vi "FromRepo.vi"(8 "error in":errorcluster, 9 "from repo cluster":T2, 10 "repository in":refnum<class "NISE_CEF_Repository.lvclass">, 11 "node in":refnum<class "Target.lvclass">) -> (0 "error out":errorcluster, 2 "repository out":refnum<class "NISE_CEF_Repository.lvclass">, 3 "node":T1)   [LabVIEW 2015, in "Target.lvclass"]
doc: "Grabs information from the Repo and stores it in the nodes."
uses:
  Target.lvclass
  <vilib>/NI/Configuration Framework/Repository/NISE_CEF_Repository.lvclass
  <vilib>/NI/Configuration Framework/Node/FromRepoCluster.ctl
  <vilib>/NI/Configuration Framework/Node/NodeRef.ctl
  <vilib>/NI/Configuration Framework/Node/NISE_CEF_Node.lvclass
  CustomDeviceRepo/CustomDeviceRepo.lvclass
  CustomDeviceRepo/CustomDeviceRepo.lvclass/CustomDeviceRepo.ctl
  Target.lvclass/Target.ctl
  CustomDeviceRepo/Read Supported Targets Properties.vi
  Write Source.vi
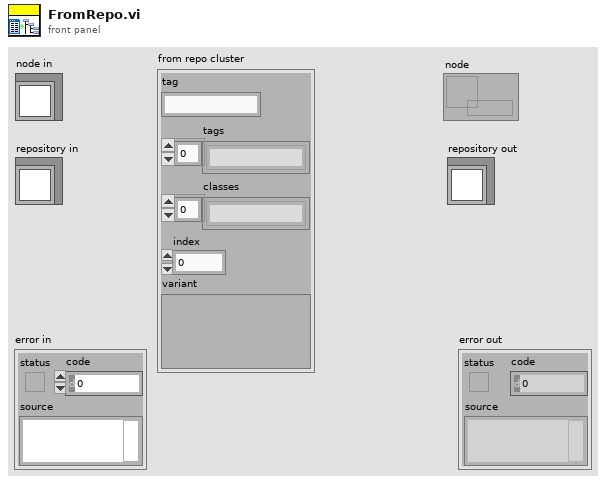
[diagram p1: front panel]
types:
  T1 = typedef "NISE_CEF_Node.lvclass/NodeRef.ctl" = refnum<data-value>
  T2 = typedef "NISE_CEF_Node.lvclass/FromRepoCluster.ctl" = cluster{"tag":string, "tags":string[], "classes":string[], "index":i32, "variant":variant}
  T3 = typedef "Source Distribution for Custom Device VI.ctl" = cluster{"Source":T4, "Real Time System Destination":string, "Supported Target":T5}[]
  T4 = typedef "Path Cluster.ctl" = cluster{"Path":path, "Path Type":enum16{"Absolute", "To Base", "To Common Doc Dir", "To Application Data Dir"}}
  T5 = typedef "Target.ctl" = enum16{"All", "Pharlap", "VxWorks", "Windows", "Linux_32_ARM", "Linux_x64", "PharlapWindows", "PharlapVxWorks", "VxWorksWindows"}
  T6 = cluster{"Source":T4, "Real Time System Destination":string, "Supported Target":T5}
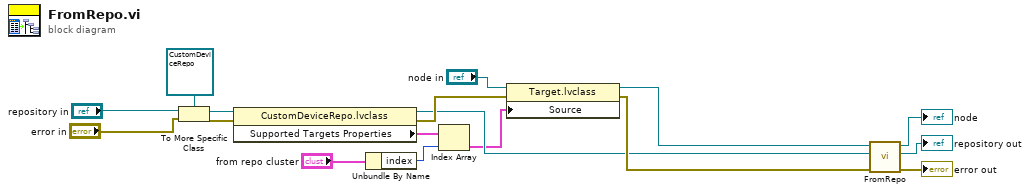
[diagram p0: block diagram]
diagram:
  n1 = To More Specific Class(target class=refnum<class "CustomDeviceRepo.lvclass"> refnum, reference="repository in", error in="error in") -> (specific class reference=w10:refnum<class "CustomDeviceRepo.lvclass">, error out=w8:errorcluster)
  n2 = property class="CustomDeviceRepo.lvclass"(reference=w10, error in=w8) -> (reference out=w2:refnum<class "CustomDeviceRepo.lvclass">, error out=w5:errorcluster, "Supported Targets Properties"=w7:T3)
  n3 = Unbundle By Name("from repo cluster") -> ("index"=w6:i32)
  n4 = Index Array(array=w7, index=w6) -> (element=w1:T6)
  n5 = property class="Target.lvclass"(reference="node in", error in=w5, "Source"=w1) -> (reference out=w3:refnum<class "Target.lvclass">, error out=w4:errorcluster)
  n6 = call-parent "FromRepo.vi"("error in"=w4, "repository in"=w2, "node in"=w3) -> ("error out"=→"error out":errorcluster, "repository out"=→"repository out":refnum<class "NISE_CEF_Repository.lvclass">, "node"=→"node":T1)  [unwired: 6 in]
